vi "Setup.vi"(11 "SessionHandler in":refnum<class "SessionHandler.lvclass">) -> (0 "error out":errorcluster, 3 "SessionHandler out":refnum<class "SessionHandler.lvclass">)   [LabVIEW 2017, in "Network Sink.lvlib" / "SessionHandler.lvclass"]
uses:
  <vilib>/gpm_packages/@cs/event-logger/Source/Network Sink/SessionHandler/SessionHandler.lvclass
  <vilib>/gpm_packages/@cs/event-logger/Source/Network Sink/SessionHandler/SessionHandler.lvclass/SessionHandler.ctl
  <vilib>/gpm_packages/@cs/Network-sink/Source/Network Interface/Network Interface/Network Interface.lvclass
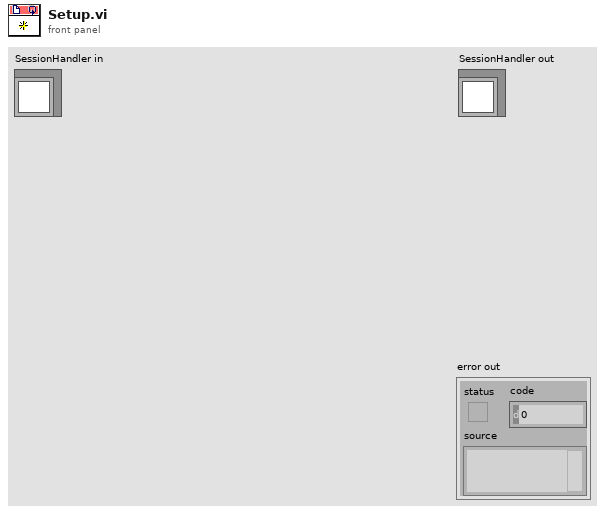
[diagram p1: front panel]
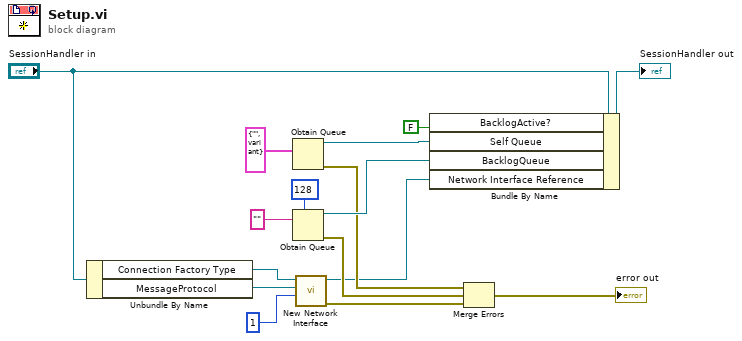
[diagram p0: block diagram]
diagram:
  n1 = Unbundle By Name("SessionHandler in") -> ("Connection Factory Type"=w1:refnum<class "IConnectionFactory.lvclass">, "MessageProtocol"=w3:refnum<class "IMessagingProtocol.lvclass">)
  n2 = Obtain Queue(element data type=cluster{"Message":string, "Data":variant} {"Message"="", "Data"=variant} ("element")) -> (queue out=w14:refnum<queue>, error out=w8:errorcluster)  [unwired: 4 in, 1 out]
  n3 = Obtain Queue(max queue size (-1, unlimited)=128, element data type="") -> (queue out=w12:refnum<queue>, error out=w9:errorcluster)  [unwired: 3 in, 1 out]
  n4 = call <vilib>:"New Network Interface.vi"("Max Number of Connections to Create (1)"=1 ("Max Number of Connections"), "MessageProtocol"=w3, "Connection Factory Type"=w1) -> ("error out"=w6:errorcluster, "Network Interface Reference"=w5:refnum<data-value>)  [unwired: 7 in]
  n5 = Bundle By Name(cluster="SessionHandler in", "BacklogActive?"=FALSE, "Self Queue"=w14, "BacklogQueue"=w12, "Network Interface Reference"=w5) -> (→"SessionHandler out":refnum<class "SessionHandler.lvclass">)
  n6 = Merge Errors(w8, w9, w6) -> (→"error out":errorcluster)
